vi "Send log data.vi"(11 "signal in":waveform(dbl)) -> ()   [LabVIEW 2019, in "HELPER LOOP ACQ.lvlib"]
uses:
  HELPER LOOP ACQ.lvlib
  <vilib>/measure/NI_MAPro.lvlib
  <vilib>/measure/mascope.llb/Amplitude and Levels 1 chan.vi
  <vilib>/measure/matone.llb/Extract Single Tone Information 1 Chan.vi
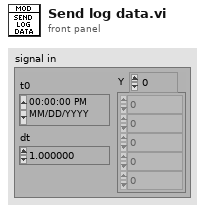
[diagram p1: front panel]
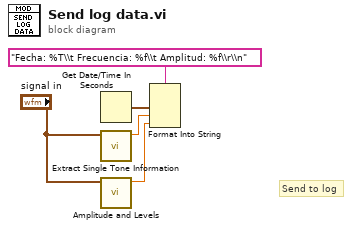
[diagram p0: block diagram]
diagram:
  # "Send to log"
  n1 = Get Date/Time In Seconds() -> (seconds since 1Jan1904=w3:timestamp)
  n2 = call-poly <vilib>:"Extract Single Tone Information.vi"("time signal in"="signal in") -> ("detected frequency"=w4:dbl)  [unwired: 5 in, 5 out]
  n3 = call-poly <vilib>:"Amplitude and Levels.vi"("signal in"="signal in") -> ("amplitude"=w5:dbl)  [unwired: 7 in, 3 out]
  n4 = Format Into String(format string="Fecha: %T\\t Frecuencia: %f\\t Amplitud: %f\\r\\n", w3, w4, w5) -> ()  [unwired: 2 in, 2 out]
